vi "HRANDFIELD.vi"(6 "with values?":bool, 8 "error in (no error)":errorcluster, 9 "count":i64, 10 "key":string, 11 "Redis Client in":refnum<class "Redis Client.lvclass">) -> (0 "error out":errorcluster, 1 "found?":bool, 2 "RESP3 Value":variant, 3 "Redis Client out":refnum<class "Redis Client.lvclass">)   [LabVIEW 2019, in "Redis Client for LabVIEW.lvlib" / "Redis Client.lvclass"]
uses:
  Redis Client.lvclass
  RESP3 for LabVIEW/RESP3/RESP3.lvlib
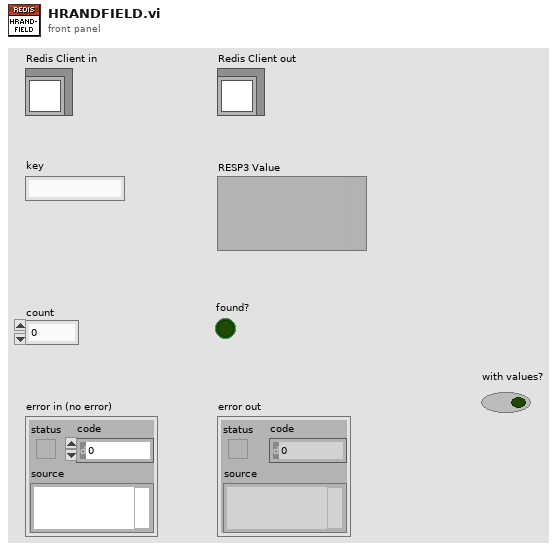
[diagram p1: front panel]
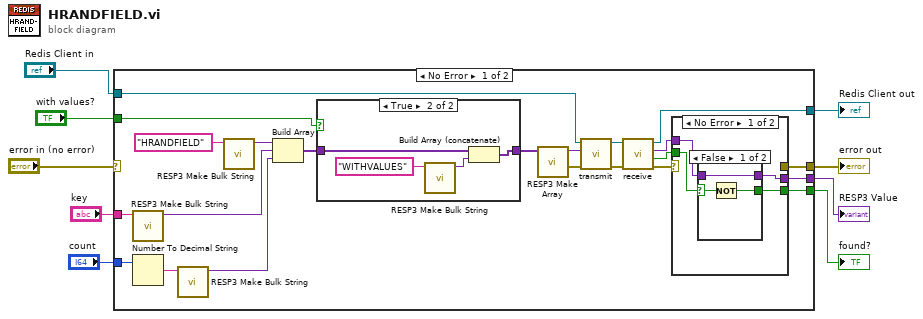
[diagram p0: block diagram]
diagram:
  n1 = case shown="No Error" "error in (no error)" {
    selector: "error in (no error)" -> [_ w46]
    tunnel: [w18 w46] -> w8
    tunnel: "Redis Client in" -> [w31 w45]
    tunnel: [w29 w45] -> w6
    tunnel: "key" -> [w26 _]
    tunnel: "count" -> [w25 _]
    tunnel: [w17 _] -> w3
    tunnel: [w14 _] -> w2
    tunnel: "with values?" -> [w13 _]
    frame No Error {
      n2 = call "RESP3 Make Bulk String.vi"("String"=w26) -> ("RESP3 Value out"=w23:variant)  [unwired: 9 in, 1 out]
      n3 = Number To Decimal String(number=w25) -> (decimal integer string=w10:string)  [unwired: 1 in]
      n4 = call "RESP3 Make Bulk String.vi"("String"=w10) -> ("RESP3 Value out"=w22:variant)  [unwired: 9 in, 1 out]
      n5 = call "RESP3 Make Bulk String.vi"("String"="HRANDFIELD" ("string in")) -> ("RESP3 Value out"=w24:variant)  [unwired: 9 in, 1 out]
      n6 = Build Array(w24, w23, w22) -> (w12:variant[])
      n7 = case shown="True" w13 {
        tunnel: w12 -> [w32 w34]
        tunnel: [w32 w33] -> w11
        frame False {
        }
        frame True {
          n8 = call "RESP3 Make Bulk String.vi"("String"="WITHVALUES") -> ("RESP3 Value out"=w35:variant)  [unwired: 9 in, 1 out]
          n9 = Build Array (concatenate)(w34, w35) -> (w33:variant[])
        }
      }
      n10 = call "RESP3 Make Array.vi"("RESP3 Values in"=w11) -> ("error out"=w20:errorcluster, "RESP3 Value out"=w21:variant)  [unwired: 9 in]
      n11 = call-dynamic "transmit.vi"("error in (no error)"=w20, "RESP3 Value"=w21, "Redis Client in"=w31) -> ("error out"=w28:errorcluster, "Redis Client out"=w30:refnum<class "Redis Client.lvclass">)  [unwired: 7 in]
      n12 = call-dynamic "receive.vi"("error in (no error)"=w28, "Redis Client in"=w30) -> ("error out"=w16:errorcluster, "timed out?"=w15:bool, "RESP3 Value"=w19:variant, "Redis Client out"=w29:refnum<class "Redis Client.lvclass">)  [unwired: 6 in]
      n13 = case shown="No Error" w16 {
        selector: w16 -> [_ w44]
        tunnel: w19 -> [w40 _]
        tunnel: [_ w44] -> w18
        tunnel: [w39 _] -> w17
        tunnel: w15 -> [w38 _]
        tunnel: [w37 _] -> w14
        frame No Error {
          n14 = case shown="False" w38 {
            selector: w38 -> [w41 _]
            tunnel: w40 -> [w42 _]
            tunnel: [w43 _] -> w39
            tunnel: [w42 _] -> w37
            frame False {
              n15 = Not(x=w41) -> (.not. x?=w43:bool)
            }
            frame True {
            }
          }
        }
        frame Error {
        }
      }
    }
    frame Error {
    }
  }
  "error out" <- w8
  "Redis Client out" <- w6
  "RESP3 Value" <- w2
  "found?" <- w3
